vi "ScanHarmonics.vi"() -> ()   [LabVIEW 2016]
uses:
  <vilib>/Instr/_visa.llb/VISA Configure Serial Port (Instr).vi
panel:
  out "Start Time":string
  out "RoiSum":dbl=24008.0
  in  "Main UI":T1(tab)=enum."Collect Data"
  in  "Get Position":bool
  in  "Set Zero Position":bool
  in  "Move to Target":bool
  in  "Arduino USB Port":refnum<visa-resource-name>="COM3"
  in  "Target Motor Position":i32
  out "Current Position":string="0\r\n"
  in  "Reset Arduino":bool
  out "Settings":T2={"Range"=3520, "cftfak"=39321856, "RoiMin"=0, "RoiMax"=3520, "#Regions"=0, "Caluse"=1, "Calpoints"=0, "Param"=0, "Offset"=0, "Xdim"=0, "bitshift"=0, "Active"=1, "Roipreset"=10.0, "dummy1"=0.0, "dummy2"=0.0, "dummy3"=0.0} {"dummy3" format="%.2f"; "dummy2" format="%.2f"; "bitshift" format="%.0x"; "Active" format="%.0x"; "Offset" format="%.0x"; "Param" format="%.0x"; "dummy1" format="%.2f"; "Roipreset" format="%.2f"; "cftfak" format="%.0x"}
  in  "Maximum Scan\nPosition":dbl=3000.0
  out "Harmonics":cluster{"Y":dbl[], "Y":dbl[]}[](graph)=[{"Y"=[200.0, 300.0, 400.0, 500.0, 600.0, 700.0, 800.0, 900.0, 1000.0, 1100.0, 1200.0, 1300.0, 1400.0, 1500.0, 1600.0, 1700.0, 1800.0, 1900.0, 2000.0, 2100.0, 2200.0, 2300.0, 2400.0, 2500.0, 2600.0, 2700.0, 2800.0, 2900.0, 3000.0, 3100.0, 3200.0, 3300.0], "Y"=[0.0, 24008.0, 24008.0, 24008.0, 24008.0, 24008.0, 24008.0, 24008.0, 24008.0, 24008.0, 24008.0, 24008.0, 24008.0, 24008.0, 24008.0, 24008.0, 24008.0, 24008.0, 24008.0, 24008.0, 24008.0, 24008.0, 24008.0, 24008.0, 24008.0, 24008.0, 24008.0, 24008.0, 24008.0, 24008.0, 24008.0, 24008.0]}]
  in  "Start Scan":bool
  out "Spectrum":u32[](graph)
  in  "State":T3(ring)=enum."Move Grating"
  out "Grating Position":i16=3300
  in  "Step Size":i32=100
  in  "Sweeps":i32
  out "CHN Status":T4={"Started"=0, "Maxval"=3001, "Runtime"=0.018000000000000002, "Fifo full"=0.0, "TotalSum"=24008.0, "RoiSum"=24008.0, "Roirate"=0.0, "Sweeps"=3001.0, "Starts"=3001.0, "Dummy"=0.0} {"Dummy" format="%.2f"; "Starts" format="%.2f"; "Sweeps" format="%.2f"; "Roirate" format="%.2f"; "RoiSum" format="%.2f"; "TotalSum" format="%.2f"; "Fifo full" format="%.2f"; "Runtime" format="%.2f"}
  in  "Photoelectron Spectra Destination":path=path "C:/Users/cj09d/Desktop/SpectraTest/Today"
  out "Halt Confirmation":string="OK"
  out "MCSADat Error":i32
  in  "Spectrum #":i32
  out "Arduino Response":string="1600\r\n"
  out "Sent Message":string="M003300#"
  in  "Stop":bool
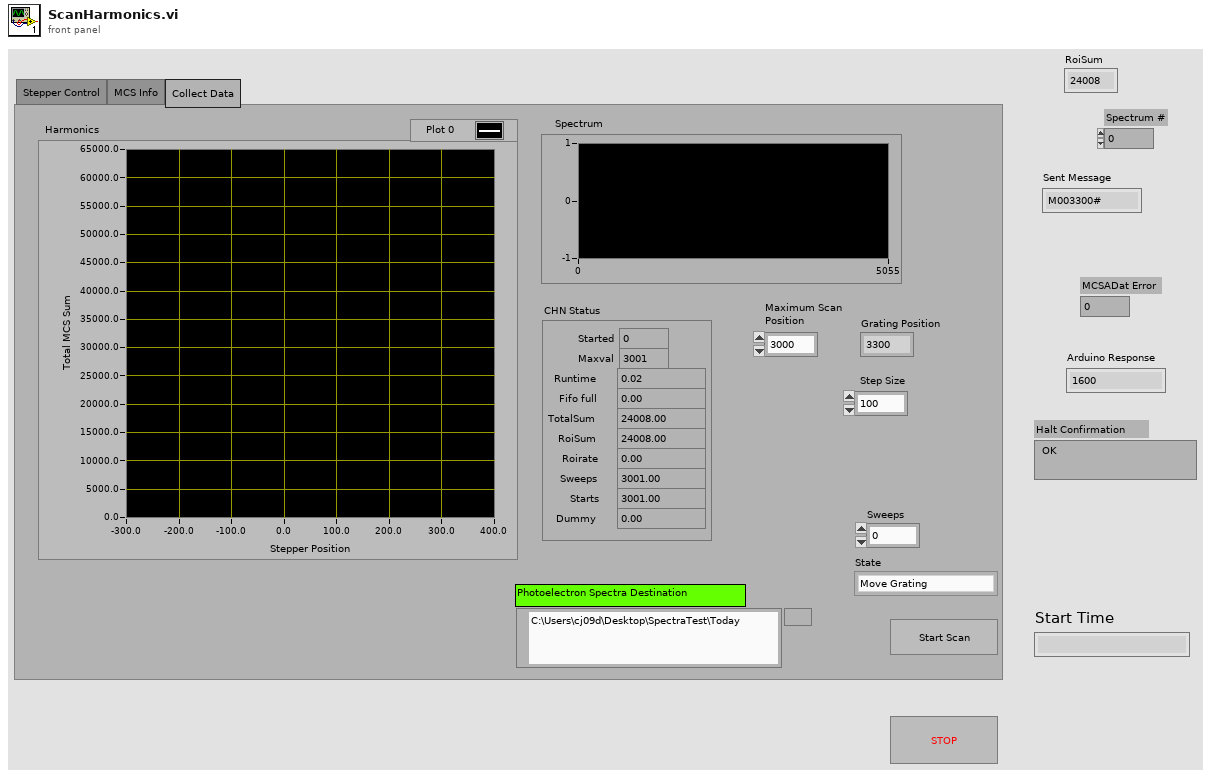
[diagram p1: front panel]
types:
  T1 = enum32{"Stepper Control", "MCS Info", "Collect Data"}
  T2 = cluster{"Range":i32, "cftfak":i32, "RoiMin":i32, "RoiMax":i32, "#Regions":i32, "Caluse":i32, "Calpoints":i32, "Param":i32, "Offset":i32, "Xdim":i32, "bitshift":i32, "Active":i32, "Roipreset":dbl, "dummy1":dbl, "dummy2":dbl, "dummy3":dbl}
  T3 = enum16{"Start", "Move Grating", "Start MCS", "Collect Data", "Stop MCS", "Save Data", "Stop"}
  T4 = cluster{"Started":i32, "Maxval":u32, "Runtime":dbl, "Fifo full":dbl, "TotalSum":dbl, "RoiSum":dbl, "Roirate":dbl, "Sweeps":dbl, "Starts":dbl, "Dummy":dbl}
  T5 = enum16{"open", "replace", "create", "open or create", "replace or create", "replace or create with confirmation"}
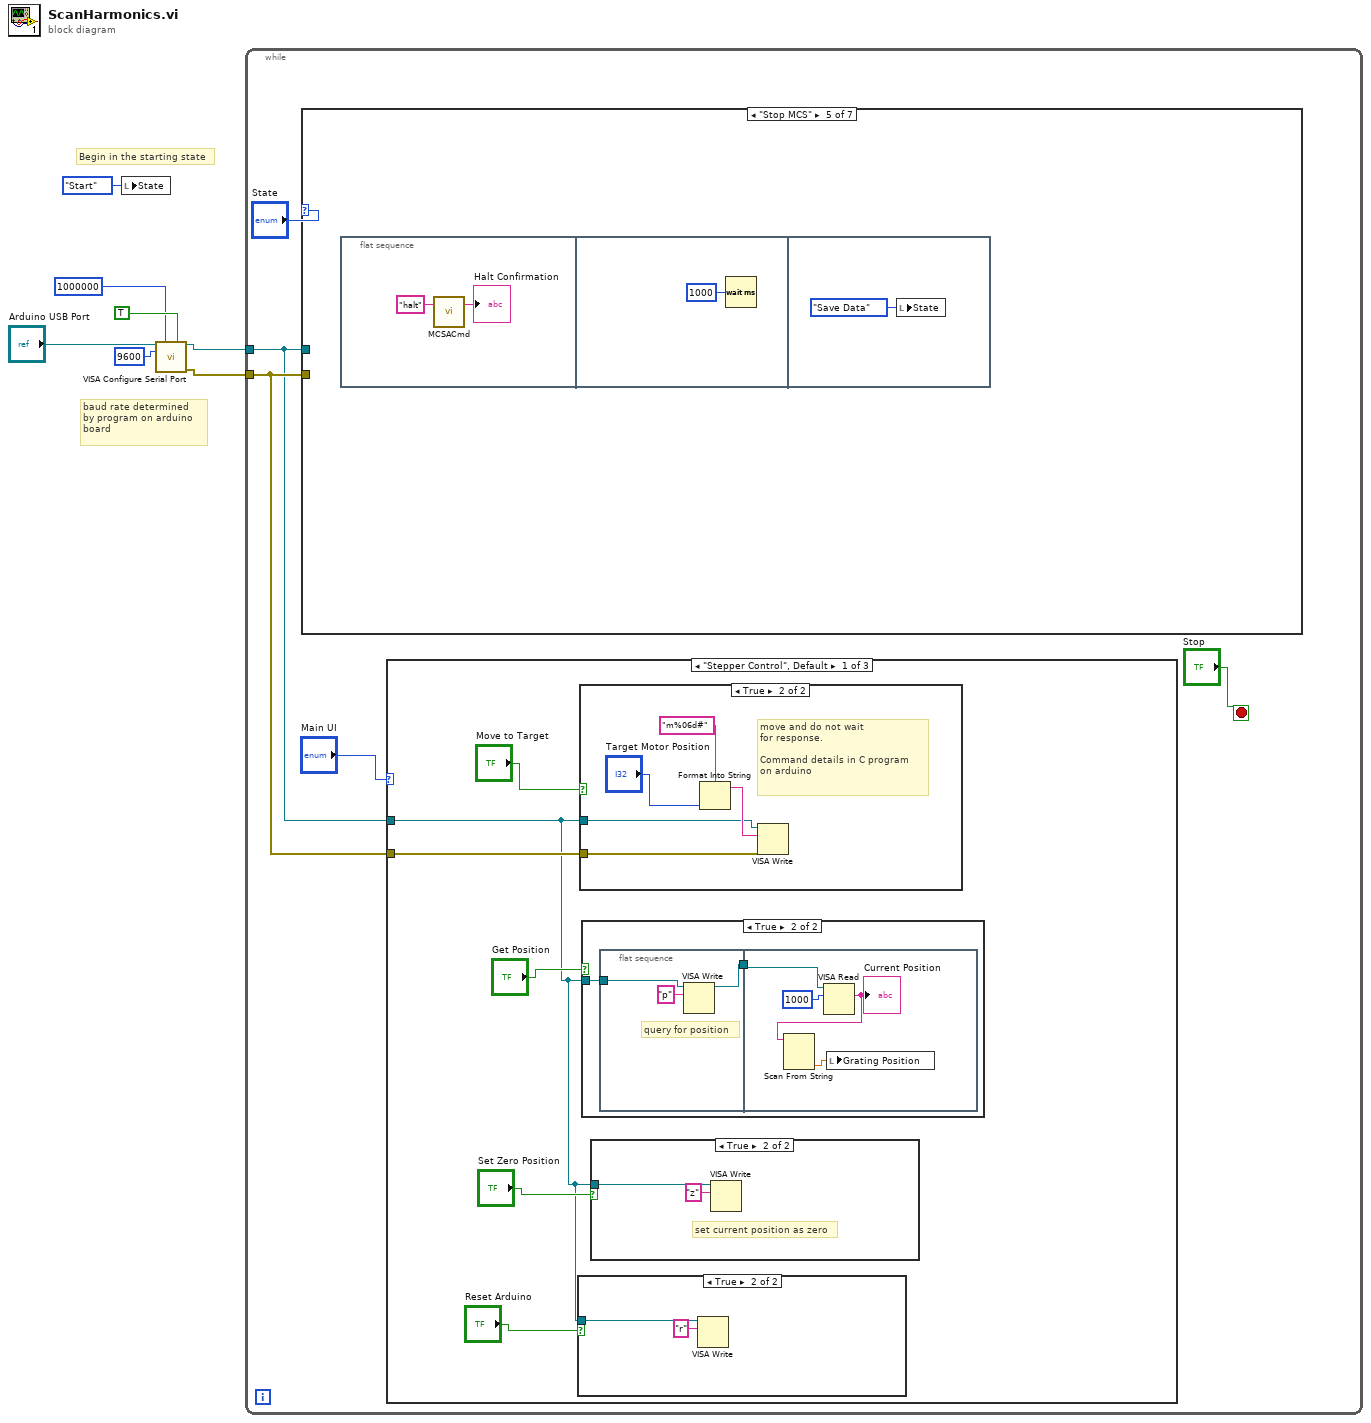
[diagram p0: block diagram]
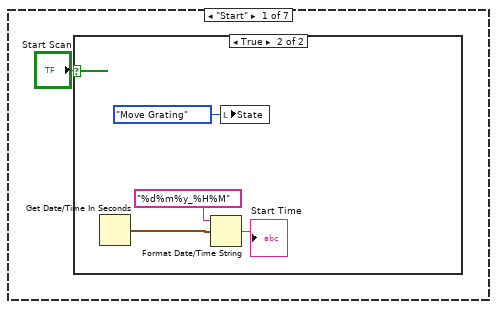
[diagram p8: hidden frame]
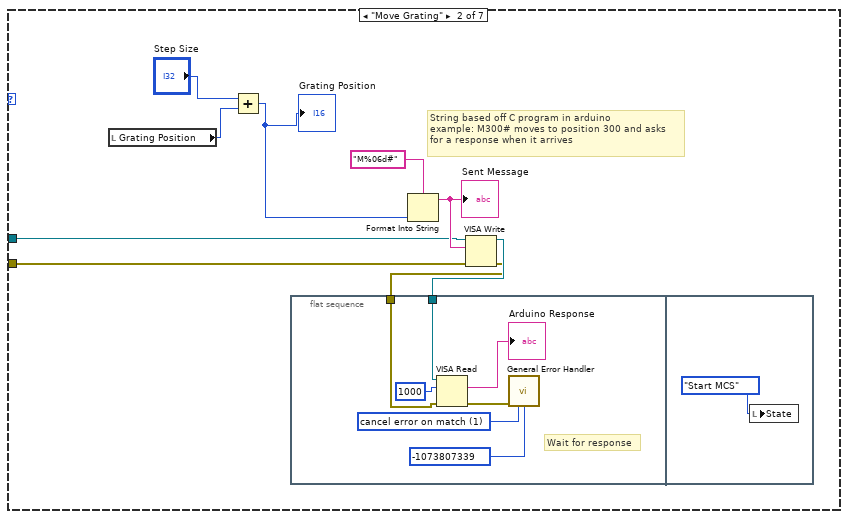
[diagram p10: hidden frame]
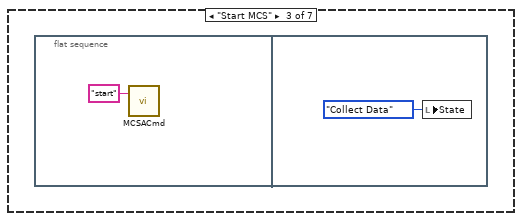
[diagram p11: hidden frame]
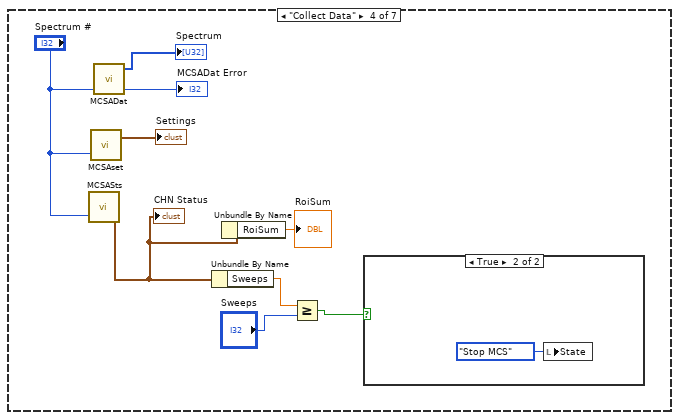
[diagram p12: hidden frame]
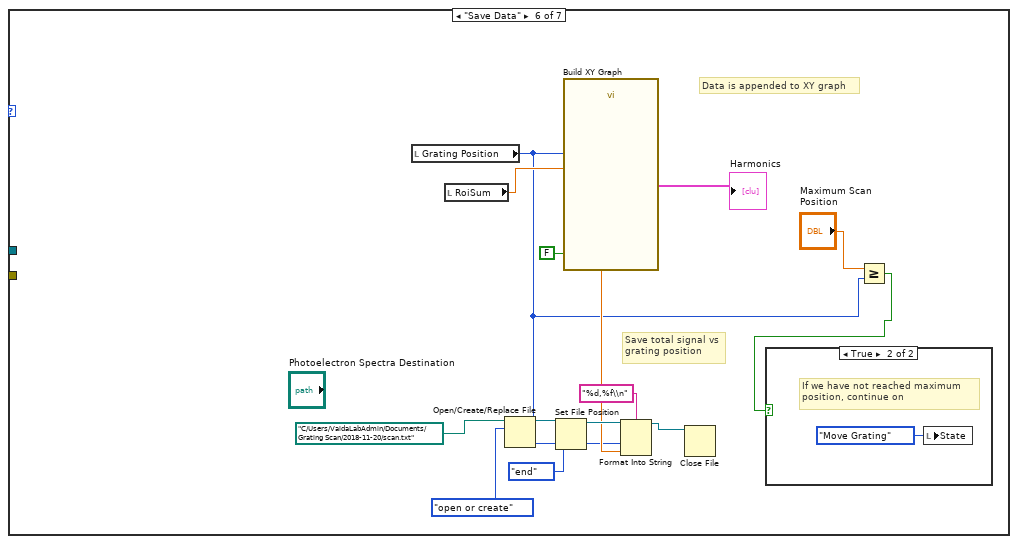
[diagram p14: hidden frame]
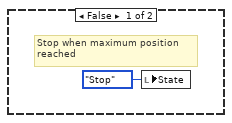
[diagram p15: hidden frame]
diagram:
  # "Begin in the starting state"
  # "baud rate determined\nby program on arduino\nboard"
  n1 = local write "State"(T3."Start" ("State")) -> ()
  n2 = call-poly "VISA Configure Serial Port"("VISA resource name"="Arduino USB Port", "timeout (10sec)"=u32 1000000, "Enable Termination\nChar (T)"=TRUE, "baud rate (9600)"=u32 9600 ("baud rate")) -> ("VISA resource name out"=w1:refnum<visa-resource-name>, "error out"=w2:errorcluster)  [unwired: 6 in, 4 out]
  n3 = while {
    tunnel: w1 -> [w9]
    tunnel: w2 -> [w10]
    stop <- "Stop" stop-if-true
    n4 = case shown="\"Stop MCS\"" "State" {
      tunnel: w9 -> [_ w48 _ _ _ _ _]
      tunnel: w10 -> [_ w47 _ _ _ _ _]
      frame "Start" {
        n5 = case shown="True" "Start Scan" {
          frame False {
          }
          frame True {
            n6 = Get Date/Time In Seconds() -> (seconds since 1Jan1904=w39:timestamp)
            n7 = Format Date/Time String(time format string (%c)="%d%m%y_%H%M", seconds (now)=w39) -> (date/time string=→"Start Time":string)  [unwired: 1 in]
            n8 = local write "State"(T3."Move Grating" ("State")) -> ()
          }
        }
      }
      frame "Move Grating" {
        # "String based off C program in arduino\nexample: M300# moves to position 300 and asks\nfor a response when it arrives"
        n9 = local read "Grating Position"() -> (w45:i16)
        n10 = Add(x="Step Size", y=w45) -> (x+y=w42:i32)
        "Grating Position" <- w42
        n11 = flat-sequence {
          tunnel: w44 -> [w52]
          tunnel: w43 -> [w51]
          frame #0 {
            w55 = 1 items=["no exception", "cancel error on match", "set error on match"] ("[exception action] (none:0)")
            # "Wait for response"
            n12 = VISA Read(VISA resource name=w52, byte count=1000, error in (no error)=w51) -> (read buffer=→"Arduino Response":string, error out=w57:errorcluster)  [unwired: 2 out]
            n13 = call <vilib>:"General Error Handler.vi"("error in (no error)"=w57, "[exception action] (none:0)"=w55, "[exception code]"=-1073807339) -> ()  [unwired: 8 in, 5 out]
          }
          frame #1 {
            n14 = local write "State"(T3."Start MCS" ("State")) -> ()
          }
        }
        n15 = Format Into String(format string="M%06d#", w42) -> (resulting string=w49:string)  [unwired: 2 in, 1 out]
        "Sent Message" <- w49
        n16 = VISA Write(VISA resource name=w48, write buffer=w49, error in (no error)=w47) -> (VISA resource name out=w44:refnum<visa-resource-name>, error out=w43:errorcluster)  [unwired: 1 out]
      }
      frame "Start MCS" {
        n17 = flat-sequence {
          frame #0 {
            n18 = call "MCSACmd.vi"("Command"="start") -> ()  [unwired: 2 in, 1 out]
          }
          frame #1 {
            n19 = local write "State"(T3."Collect Data" ("State")) -> ()
          }
        }
      }
      frame "Collect Data" {
        n20 = call "MCSASts.vi"("CHN #"="Spectrum #") -> ("CHN Status"=w62:T4)  [unwired: 1 in, 1 out]
        "CHN Status" <- w62
        n21 = call "MCSAset.vi"("Spect #"="Spectrum #") -> ("Settings"=→"Settings":T2)  [unwired: 1 in, 1 out]
        n22 = call "MCSADat.vi"("Spectrum #"="Spectrum #") -> ("MCSADat Error"=→"MCSADat Error":i32, "Data"=→"Spectrum":u32[])  [unwired: 2 in, 1 out]
        n23 = Unbundle By Name(w62) -> ("Sweeps"=w65:dbl)
        n24 = Unbundle By Name(w62) -> ("RoiSum"=→"RoiSum":dbl)
        n25 = Greater Or Equal?(x=w65, y="Sweeps") -> (x >= y?=w63:bool)
        n26 = case shown="True" w63 {
          frame False {
            # "Do nothing, continue\ncollecting data"
          }
          frame True {
            n27 = local write "State"(T3."Stop MCS" ("State")) -> ()
          }
        }
      }
      frame "Stop MCS" {
        n28 = flat-sequence {
          frame #0 {
            n29 = call "MCSACmd.vi"("Command"="halt") -> ("Response"=→"Halt Confirmation":string)  [unwired: 2 in]
          }
          frame #1 {
            n30 = Wait (ms)(milliseconds to wait=u32 1000) -> ()  [unwired: 1 out]
          }
          frame #2 {
            n31 = local write "State"(T3."Save Data" ("State")) -> ()
          }
        }
      }
      frame "Save Data" {
        # "Data is appended to XY graph"
        # "Save total signal vs\ngrating position"
        n32 = local read "Grating Position"() -> (w77:i16)
        n33 = local read "RoiSum"() -> (w82:dbl)
        n34 = Open/Create/Replace File(file path (use dialog)=path "C:/Users/VaidaLabAdmin/Documents/Grating Scan/2018-11-20/scan.txt", operation (0:open)=T5."open or create") -> (refnum out=w85:refnum<file>)  [unwired: 4 in, 2 out]
        n35 = Set File Position(refnum=w85, from (0:start)=enum16{"start", "end", "current"}."end") -> (refnum out=w83:refnum<file>)  [unwired: 2 in, 1 out]
        n36 = call "Build XY Graph"("Reset"=FALSE, "Y Input"=w82, "X Input"=w77) -> ("XY Graph"=→"Harmonics":cluster{"X":dbl[], "Y":dbl[]}[])  [unwired: 7 in, 1 out]
        n37 = Format Into String(format string="%d,%f\\n", initial string=w83, w77, w82) -> (resulting string=w80:refnum<file>)  [unwired: 1 in, 1 out]
        n38 = Close File(refnum=w80) -> ()  [unwired: 1 in, 2 out]
        n39 = Greater Or Equal?(x="Maximum Scan\nPosition", y=w77) -> (x >= y?=w76:bool)
        n40 = case shown="True" w76 {
          frame False {
            # "Stop when maximum position\nreached"
            n41 = local write "State"(T3."Stop" ("State")) -> ()
          }
          frame True {
            # "If we have not reached maximum\nposition, continue on"
            n42 = local write "State"(T3."Move Grating" ("State")) -> ()
          }
        }
      }
      frame "Stop", Default {
      }
    }
    n43 = case shown="\"Stepper Control\", Default" "Main UI" {
      tunnel: w10 -> [w16 _ _]
      tunnel: w9 -> [w13 _ _]
      frame "Stepper Control", Default {
        n44 = case shown="True" "Reset Arduino" {
          tunnel: w13 -> [_ w19]
          frame False {
          }
          frame True {
            n45 = VISA Write(VISA resource name=w19, write buffer="r") -> ()  [unwired: 1 in, 3 out]
          }
        }
        n46 = case shown="True" "Move to Target" {
          tunnel: w16 -> [_ w33]
          tunnel: w13 -> [_ w32]
          frame False {
          }
          frame True {
            # "move and do not wait\nfor response.\n\nCommand details in C program\non arduino"
            n47 = Format Into String(format string="m%06d#", "Target Motor Position") -> (resulting string=w35:string)  [unwired: 2 in, 1 out]
            n48 = VISA Write(VISA resource name=w32, write buffer=w35, error in (no error)=w33) -> ()  [unwired: 3 out]
          }
        }
        n49 = case shown="True" "Get Position" {
          tunnel: w13 -> [_ w23]
          frame False {
          }
          frame True {
            n50 = flat-sequence {
              tunnel: [w27] -> w24
              tunnel: w23 -> [w25]
              tunnel: w24 -> [w30]
              frame #0 {
                # "query for position"
                n51 = VISA Write(VISA resource name=w25, write buffer="p") -> (VISA resource name out=w27:refnum<visa-resource-name>)  [unwired: 1 in, 2 out]
              }
              frame #1 {
                n52 = VISA Read(VISA resource name=w30, byte count=1000) -> (read buffer=w29:string)  [unwired: 1 in, 3 out]
                "Current Position" <- w29
                n53 = Scan From String(input string=w29) -> (output 1=w28:dbl)  [unwired: 4 in, 3 out]
                n54 = local write "Grating Position"(w28) -> ()
              }
            }
          }
        }
        n55 = case shown="True" "Set Zero Position" {
          tunnel: w13 -> [_ w21]
          frame False {
          }
          frame True {
            # "set current position as zero"
            n56 = VISA Write(VISA resource name=w21, write buffer="z") -> ()  [unwired: 1 in, 3 out]
          }
        }
      }
      frame "MCS Info" {
        # "Ensure MCS6A.exe is running and that the 32/64 bit version of LabView matches the version of the MCS\nsoftware running, most setup done through that program\n\nIn particular set a Sweeps Preset under Hardware Options to be the desired sweeps + 1"
      }
      frame "Collect Data" {
        # "This state is continuously running based on the State variable\nSee large above case structure"
      }
    }
  }
